vi "HXG2_GroupInitialize.vi"(6 "Profile Name":string, 8 "error in":errorcluster) -> (0 "error out":errorcluster)   [LabVIEW 2012]
doc: "- Get reference to the table control\n- Load a profile to the table\n- Write path to the profile used in the FGV\n- Parse data for use in Programmer\n- Initialize all UI controls to F and no repeat executions"
uses:
  Modules/Programmer/HXG2programmer.ctl
  Modules/Programmer/HXG2programmerUserSelections.ctl
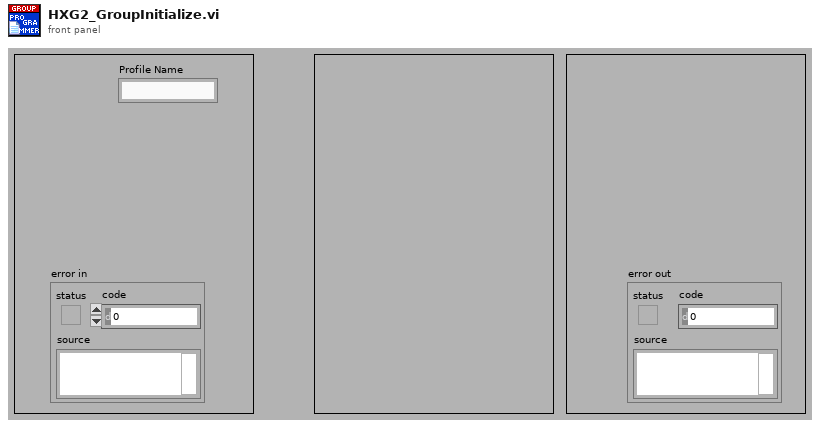
[diagram p1: front panel]
types:
  T1 = typedef "HXG2programmer.ctl" = enum16{"Write Refs", "Write Selec", "Write All", "Pass All", "React", "Write Path"}
  T2 = typedef "HXG2programmerUserSelections.ctl" = cluster{"Run Prog":bool, "Done Stop":bool, "Load Profile":bool, "Save Profile":bool, "Repeat Execution:":i32, "Start Programmer":bool, "Stop Programmer":bool}
  T3 = typedef "HXG2_ProgRefs.ctl" = cluster{"Prog. Indicator":refnum<vi>, "Table":refnum<vi>, "Save Button":refnum<vi>, "Duration Ctrl":refnum<vi>, "Run Prog":refnum<vi>}
  T4 = typedef "Programmer Step.ctl" = cluster{"Airflow (CFM)":T5, "Air Temp (°F)":T5, "Glycol Flow (lbm/hr)":T5, "Glycol Temp (°F)":T5, "Hold Time (min)":dbl, "Stability Test Time (min)":dbl, "Stability Timeout (min)":dbl, "Defrost?":bool}
  T5 = typedef "Programmer Step References.ctl" = cluster{"Setpoint":dbl, "Stability Range (±)":dbl}
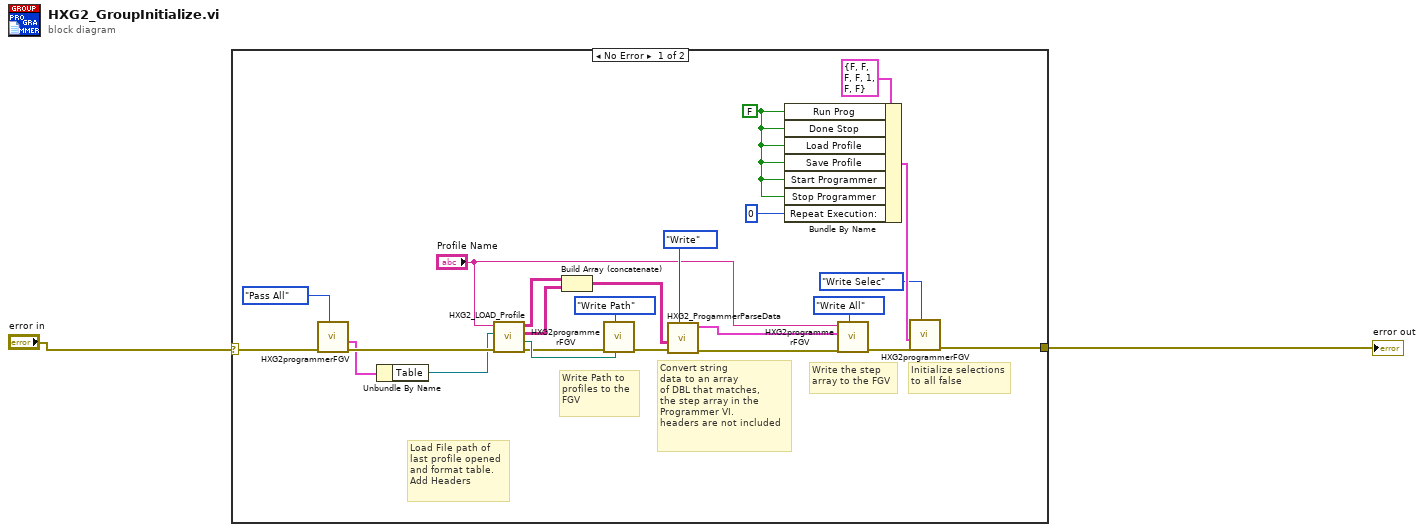
[diagram p0: block diagram]
diagram:
  n1 = case shown="No Error" "error in" {
    selector: "error in" -> [w4 w27]
    tunnel: [w3 w27] -> w1
    frame No Error {
      w9 = FALSE ("Run Programmer")
      # "Write the step\narray to the FGV"
      # "Initialize selections\nto all false"
      # "Convert string\ndata to an array\nof DBL that matches,\nthe step array in the\nProgrammer VI.\nheaders are not included"
      # "Write Path to \nprofiles to the \nFGV"
      # "Load File path of\nlast profile opened\nand format table.\nAdd Headers"
      n2 = call "HXG2programmerFGV.vi"("Programmer Ctrl"=HXG2programmer."Pass All", "error in (no error)"=w4) -> ("error out"=w8:errorcluster, "References Out"=w6:T3)  [unwired: 5 in, 3 out]
      n3 = Unbundle By Name(w6) -> ("Table"=w5:refnum<vi>)
      n4 = call "HXG2_LOAD_Profile.vi"("error in"=w8, "Table"=w5, "Programmer File"="Profile Name") -> ("error out"=w10:errorcluster, "Profile Save Path"=w12:path, "Cell Values"=w16:string[][], "Headers"=w21:string[][])  [unwired: 5 in]
      n5 = Build Array (concatenate)(w21, w16) -> (w17:string[][])
      n6 = call "HXG2programmerFGV.vi"("Path to Profile"=w12, "Programmer Ctrl"=HXG2programmer."Write Path", "error in (no error)"=w10) -> ("error out"=w14:errorcluster)  [unwired: 4 in, 4 out]
      n7 = call "HXG2_ProgammerParseData.vi"("Parse Ctrl"=enum16{"Write", "Pass"}."Write", "error in (no error)"=w14, "Table Data In"=w17) -> ("error out"=w15:errorcluster, "Step Array Out"=w18:T4[])  [unwired: 7 in]
      n8 = Bundle By Name(cluster=T2 {"Run Prog"=FALSE, "Done Stop"=FALSE, "Load Profile"=FALSE, "Save Profile"=FALSE, "Repeat Execution:"=1, "Start Programmer"=FALSE, "Stop Programmer"=FALSE} ("User Selections In"), "Run Prog"=w9, "Done Stop"=w9, "Load Profile"=w9, "Save Profile"=w9, "Start Programmer"=w9, "Stop Programmer"=w9, "Repeat Execution:"=0) -> (w25:T2)
      n9 = call "HXG2programmerFGV.vi"("Programmer Ctrl"=HXG2programmer."Write All", "error in (no error)"=w15, "Step Array"=w18, "Profile Name"="Profile Name") -> ("error out"=w22:errorcluster)  [unwired: 3 in, 4 out]
      n10 = call "HXG2programmerFGV.vi"("Programmer Ctrl"=HXG2programmer."Write Selec", "error in (no error)"=w22, "User Selections In"=w25) -> ("error out"=w3:errorcluster)  [unwired: 4 in, 4 out]
    }
    frame Error {
    }
  }
  "error out" <- w1
